vi "Test App Error Handler is Configured for Nested Process.vi"(8 "error in (no error)":errorcluster, 11 "Rig Test In":refnum<class "Application Dev Test.lvclass">) -> (0 "error out":errorcluster, 3 "Rig Test Out":refnum<class "Application Dev Test.lvclass">)   [LabVIEW 2020, in "Application Dev Test.lvclass"]
uses:
  Application Dev Test.lvclass
  C:/Program Files (x86)/National Instruments/LabVIEW 2020/vi.lib/Astemes/LUnit/Test Case.lvclass
  source/Framework Test Suite/Mock Error Handler/Mock Error Handler.lvclass
  C:/Git/astemes-triarc-framework/source/Framework/Error Handler Interface/Error Handler Interface.lvclass
  source/Framework Test Suite/Mock Process/Mock Process.lvclass
  C:/Git/astemes-triarc-framework/source/Framework/Process/Process.lvclass
  source/Framework/Application/Application.lvclass
  source/Framework/Process/Process.lvclass/Process.ctl
  source/Framework/Application/Application.lvclass/Application.ctl
  <vilib>/Astemes/LUnit/Test Case.lvclass/Test Case.ctl
  <vilib>/Astemes/LUnit/LUnit Assertion Result.lvclass/LUnit Assertion Result.ctl
  <vilib>/Astemes/LUnit/LUnit Test Case Result.lvclass/LUnit Test Case Result.ctl
  <vilib>/Astemes/LUnit/LUnit Method Result.lvclass/LUnit Method Result.ctl
  1b0d7f43-a3d5-4dac-856a-e063cda1abe6.vi
  source/Framework/Application/Private/Add Process to Map.vi
  source/Framework/Application/Private/Start Idle Processes if Running.vi
  source/Framework/Application/Private/Throw Error If Process Already in App.vi
  source/Framework/Process/Protected/Messaging/Enqueue Message.vi
  source/Framework/Process/Public/Lifecycle/Get Lifecycle State.vi
  source/Framework/Process/Protected/SubVIs/Set Context.vi
  source/Framework/Application/Private/Retrieve Process from App.vi
  source/Framework/Application/Private/Parse Process Name.vi
  source/Framework/Application/Private/Get Process from Map.vi
  <vilib>/Astemes/LUnit/Palette/Pass.vi
  <vilib>/Astemes/LUnit/Palette/Fail.vi
  <vilib>/Astemes/LUnit/Compare Variants.vi
  <vilib>/Astemes/LUnit/Describe Comparison.vi
  <vilib>/Astemes/LUnit/Set Assertion Type.vi
  source/Framework/Process/Private/SubVIs/Wait for finish.vi
  source/Framework/Process/Private/SubVIs/Set Lifecycle State.vi
  source/Framework/Process/Private/SubVIs/Handle Debug Data.vi
  <vilib>/Utility/error.llb/Clear Errors.vi
  source/Framework/Process/Public/Lifecycle/Leave Process Loop.vi
  source/Framework/Process/Protected/Messaging/Request Message.vi
  <vilib>/AdvancedString/Delimited String to 1D String Array.vi
  <vilib>/Astemes/LUnit/Add test result.vi
  <vilib>/Astemes/LUnit/LUnit Write Passed.vi
  <vilib>/Astemes/LUnit/LUnit Write Message.vi
  <vilib>/Astemes/LUnit/LUnit Write Description.vi
  <vilib>/Astemes/LUnit/Variant to string.vi
  <vilib>/Astemes/LUnit/LUnit Write Assertion Type.vi
  source/Framework/Logging/Log Debug.vi
  <vilib>/AdvancedString/1D String Array to Delimited String.vi
  <vilib>/Utility/High Resolution Relative Seconds.vi
  source/Framework/Process/Private/SubVIs/Enqueue Request Message.vi
  <vilib>/Astemes/LUnit/LUnit Record Assertion Result.vi
  <vilib>/Astemes/LUnit/LUnit Aggregate Assertion Results.vi
  <vilib>/Astemes/LUnit/Assertion Result/LUnit Read Status.vi
  <vilib>/Astemes/LUnit/LUnit Read Message.vi
  <vilib>/Astemes/LUnit/LUnit Read Description.vi
  <vilib>/Astemes/LUnit/Method Result/LUnit Merge Status.vi
  <vilib>/Astemes/LUnit/LUnit Concatenate result strings.vi
  <vilib>/Utility/error.llb/Error Cluster From Error Code.vi
  source/Framework/Process/Public/Read Name.vi
  source/Framework/Process/Private/SubVIs/Wait for Response Message.vi
  <vilib>/Utility/Data Type/Get Type Information.vi
  <vilib>/Utility/LVClass/Get LV Class Name.vi
  source/Framework/Process/Process.lvclass
  <vilib>/Astemes/LUnit/LUnit Assertion Result.lvclass
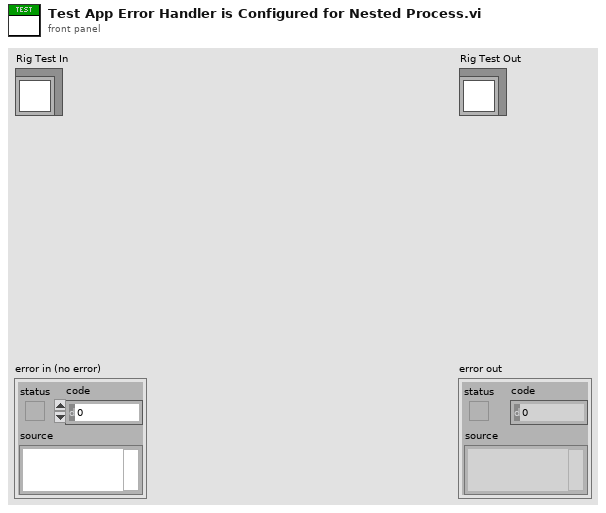
[diagram p1: front panel]
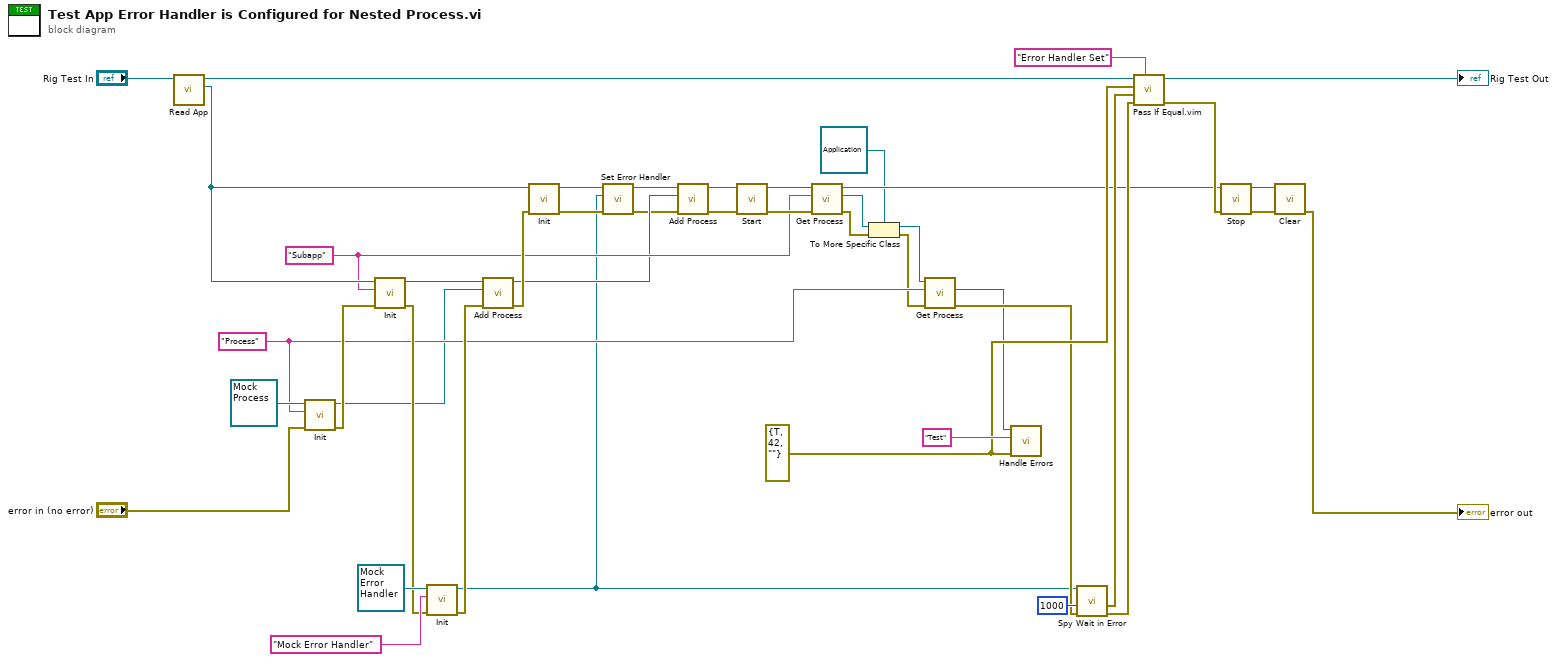
[diagram p0: block diagram]
diagram:
  w11 = "Subapp" ("Name")
  w31 = errorcluster {"status"=TRUE, "code"=42, "source"=""} ("error in (no error)")
  w26 = "Process" ("Name")
  n1 = call "Read App.vi"("Application Test In"="Rig Test In") -> ("App out"=w18:refnum<class "Application.lvclass">, "Application Test Out"=w40:refnum<class "Application Dev Test.lvclass">)  [unwired: 8 in, 1 out]
  n2 = call-dynamic "Init.vi"("error in (no error)"="error in (no error)", "Name"=w26, "Mock Process In"=refnum<class "Mock Process.lvclass"> refnum ("Mock Process.lvclass")) -> ("error out"=w35:errorcluster, "Mock Process Out"=w24:refnum<class "Mock Process.lvclass">)  [unwired: 7 in]
  n3 = call-dynamic "Init.vi"("error in (no error)"=w35, "Name"=w11, "Process In"=w18) -> ("error out"=w34:errorcluster, "Process Out"=w43:refnum<class "Application.lvclass">)  [unwired: 7 in]
  n4 = call-dynamic "Init.vi"("error in (no error)"=w34, "Name"="Mock Error Handler", "Mock Error Handler In"=refnum<class "Mock Error Handler.lvclass"> refnum ("Mock Error Handler.lvclass")) -> ("error out"=w38:errorcluster, "Mock Error Handler Out"=w1:refnum<class "Mock Error Handler.lvclass">)  [unwired: 7 in]
  n5 = call "Add Process.vi"("error in (no error)"=w38, "Process"=w24, "Application In"=w43) -> ("error out"=w14:errorcluster, "Application Out"=w6:refnum<class "Application.lvclass">)  [unwired: 7 in]
  n6 = call-dynamic "Init.vi"("error in (no error)"=w14, "Process In"=w18) -> ("error out"=w13:errorcluster, "Process Out"=w3:refnum<class "Application.lvclass">)  [unwired: 8 in]
  n7 = call "Set Error Handler.vi"("error in (no error)"=w13, "Error Handler"=w1, "Process In"=w3) -> ("error out"=w4:errorcluster, "Process Out"=w2:refnum<class "Application.lvclass">)  [unwired: 7 in]
  n8 = call "Add Process.vi"("error in (no error)"=w4, "Process"=w6, "Application In"=w2) -> ("error out"=w23:errorcluster, "Application Out"=w20:refnum<class "Application.lvclass">)  [unwired: 7 in]
  n9 = call "Start.vi"("error in (no error)"=w23, "Process In"=w20) -> ("error out"=w21:errorcluster, "Process Out"=w19:refnum<class "Application.lvclass">)  [unwired: 7 in, 1 out]
  n10 = call "Get Process.vi"("error in (no error)"=w21, "Process Name"=w11, "Application In"=w19) -> ("error out"=w8:errorcluster, "App Process"=w9:refnum<class "Process.lvclass">, "Application Out"=w12:refnum<class "Application.lvclass">)  [unwired: 6 in]
  n11 = To More Specific Class(target class=refnum<class "Application.lvclass"> refnum ("Rig Out"), reference=w9, error in=w8) -> (specific class reference=w5:refnum<class "Application.lvclass">, error out=w7:errorcluster)
  n12 = call "Get Process.vi"("error in (no error)"=w7, "Process Name"=w26, "Application In"=w5) -> ("error out"=w27:errorcluster, "App Process"=w25:refnum<class "Process.lvclass">)  [unwired: 6 in, 1 out]
  n13 = call-dynamic "Handle Errors.vi"("error in (no error)"=w31, "Location"="Test", "Process In"=w25) -> ()  [unwired: 7 in, 2 out]
  n14 = call "Spy Wait in Error.vi"("error in (no error)"=w27, "timeout in ms (-1)"=1000, "Mock Error Handler In"=w1) -> ("error out"=w29:errorcluster, "Errors"=w30:errorcluster)  [unwired: 4 in, 3 out]
  n15 = call "Pass If Equal.vim"("Description"="Error Handler Set", "error in (no error)"=w29, "Actual"=w30, "Expected"=w31, "LUnit Test Case In"=w40) -> ("error out"=w16:errorcluster, "LUnit Test Case Out"=→"Rig Test Out":refnum<class "Application Dev Test.lvclass">)  [unwired: 5 in]
  n16 = call "Stop.vi"("error in (no error)"=w16, "Process In"=w12) -> ("error out"=w17:errorcluster, "Process Out"=w22:refnum<class "Application.lvclass">)  [unwired: 7 in, 1 out]
  n17 = call-dynamic "Clear.vi"("error in (no error)"=w17, "Application In"=w22) -> ("error out"=→"error out":errorcluster)  [unwired: 9 in]
